vi "PausePump.vi"(8 "error in (no error)":errorcluster, 11 "VISA Refnum in":refnum<visa-resource-name>) -> (0 "error out":errorcluster, 3 "VISA Refnum out":refnum<visa-resource-name>)   [LabVIEW 2020]
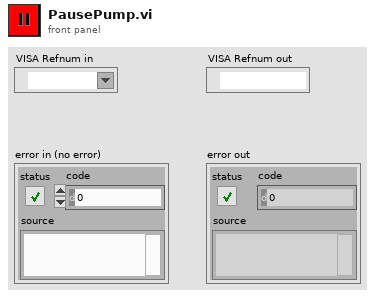
[diagram p1: front panel]
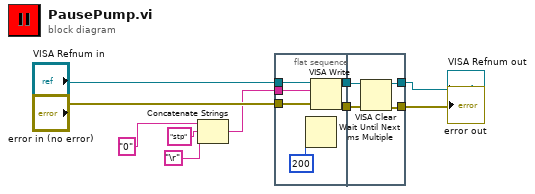
[diagram p0: block diagram]
diagram:
  n1 = Concatenate Strings("0" ("string"), "stp" ("string"), "\r") -> (w3:string)
  n2 = flat-sequence {
    tunnel: w3 -> [w16]
    tunnel: "VISA Refnum in" -> [w13]
    tunnel: "error in (no error)" -> [w12]
    tunnel: [w15] -> w10
    tunnel: [w14] -> w9
    tunnel: [w20] -> w7
    tunnel: [w17] -> w6
    tunnel: w10 -> [w19]
    tunnel: w9 -> [w18]
    frame #0 {
      n3 = Wait Until Next ms Multiple(millisecond multiple=u32 200) -> ()  [unwired: 1 out]
      n4 = VISA Write(VISA resource name=w13, write buffer=w16, error in (no error)=w12) -> (VISA resource name out=w15:refnum<visa-resource-name>, error out=w14:errorcluster)  [unwired: 1 out]
    }
    frame #1 {
      n5 = VISA Clear(VISA resource name=w19, error in (no error)=w18) -> (VISA resource name out=w17:refnum<visa-resource-name>, error out=w20:errorcluster)
    }
  }
  "error out" <- w7
  "VISA Refnum out" <- w6
